vi "Send Get Geo Codes.vi"(7 "Message Priority (Normal)":T2=enum."Normal", 8 "error in (no error)":errorcluster, 9 "Country":T1=enum."Germany", 10 "City Name":string, 11 "Message Enqueuer":refnum<class "Message Enqueuer.lvclass">) -> (0 "error out":errorcluster, 3 "Message Enqueuer out":refnum<class "Message Enqueuer.lvclass">)   [LabVIEW 2025, in "Geocoding Actor.lvlib" / "Get Geo Codes Msg.lvclass"]
doc: "This VI sends the message to an actor."
uses:
  Get Geo Codes Msg.lvclass
  <vilib>/ActorFramework/Message Enqueuer/Message Enqueuer.lvclass
  <vilib>/ActorFramework/Message Enqueuer/Message Priority.ctl
  Geocoding/Country.ctl
  C:/Program Files (x86)/National Instruments/LabVIEW 2025/vi.lib/ActorFramework/Message/Message.lvclass
  Get Geo Codes Msg.lvclass/Get Geo Codes Msg.ctl
  <vilib>/ActorFramework/Message Enqueuer/Message Enqueuer.lvclass/Message Enqueuer.ctl
  <vilib>/ActorFramework/Message Priority Queue/Priority Enqueue.vi
  Geocoding/Geocoding.lvclass
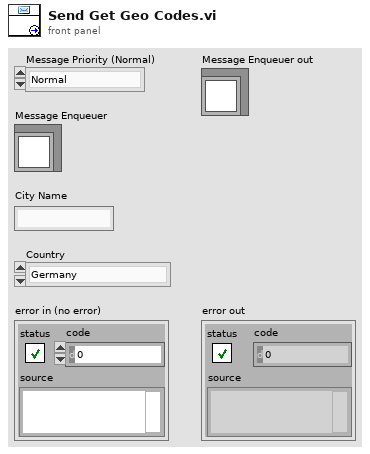
[diagram p1: front panel]
types:
  T1 = typedef "Geocoding Actor.lvlib/Geocoding.lvclass/Country.ctl" = enum16{"Austria", "Germany", "Switzerland"}
  T2 = typedef "Actor Framework.lvlib/Message Enqueuer.lvclass/Message Priority.ctl" = enum16{"Low", "Normal", "High"}
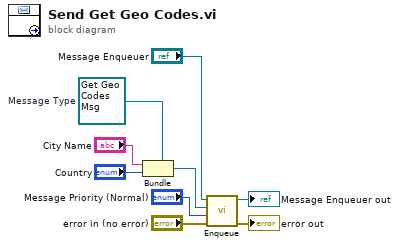
[diagram p0: block diagram]
diagram:
  w3 = refnum<class "Get Geo Codes Msg.lvclass"> refnum  # Message Type
  n1 = Bundle(cluster=w3, "City Name", "Country") -> (w4:refnum<class "Get Geo Codes Msg.lvclass">)
  n2 = call <vilib>:"Enqueue.vi"("error in (no error)"="error in (no error)", "Message Priority (Normal)"="Message Priority (Normal)", "Message"=w4, "Message Enqueuer in"="Message Enqueuer") -> ("error out"=→"error out":errorcluster, "Message Enqueuer out"=→"Message Enqueuer out":refnum<class "Message Enqueuer.lvclass">)  [unwired: 6 in]
